vi "max pwm skrecanie jazda.vi"(9 "max pwm skrecanie":i32, 10 "X axis":i32) -> (3 "y":i32)   [LabVIEW 2014]
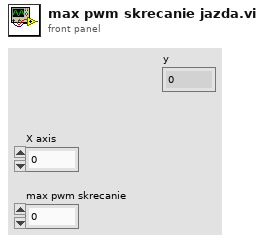
[diagram p1: front panel]
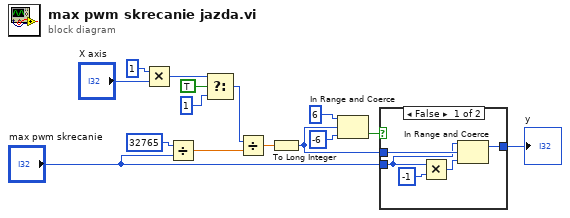
[diagram p0: block diagram]
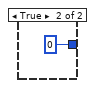
[diagram p2: hidden frame]
diagram:
  n1 = Multiply(x=1, y="X axis") -> (x*y=w10:i32)
  n2 = Divide(x=32765 ("y"), y="max pwm skrecanie") -> (x/y=w11:dbl)
  n3 = Select(t=w10, s=TRUE, f=1) -> (s? t:f=w6:i32)
  n4 = Divide(x=w6, y=w11) -> (x/y=w4:dbl)
  n5 = To Long Integer(number=w4) -> (32bit integer=w8:i32)
  n6 = In Range and Coerce(upper limit=6 ("y"), x=w8, lower limit=-6 ("y")) -> (In Range?=w7:bool)  [unwired: 1 out]
  n7 = case shown="False" w7 {
    tunnel: [w20 0 ("y")] -> w14
    tunnel: w8 -> [w19 _]
    tunnel: "max pwm skrecanie" -> [w16 _]
    frame False {
      n8 = Multiply(x=w16, y=-1) -> (x*y=w18:i32)
      n9 = In Range and Coerce(upper limit=w16, x=w19, lower limit=w18) -> (coerced(x)=w20:i32)  [unwired: 1 out]
    }
    frame True {
    }
  }
  "y" <- w14
